vi "TEST User Events XControl.vi"() -> ()   [LabVIEW 2011]
doc: "This tests and XControl that implements the generation of User Events in an X Control that are then passed to the parent VI to be handled with dynamic registration.\n\nAAL 9/09"
uses:
  XControlUserEvents.xctl
panel:
  in  "XControlUserEvents":string(xcontrol)
  in  "stop":bool
  out "Output":string
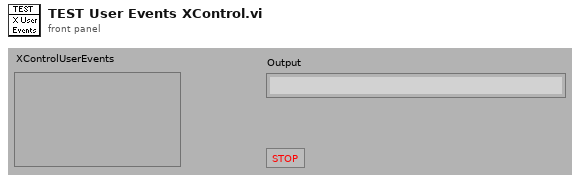
[diagram p1: front panel]
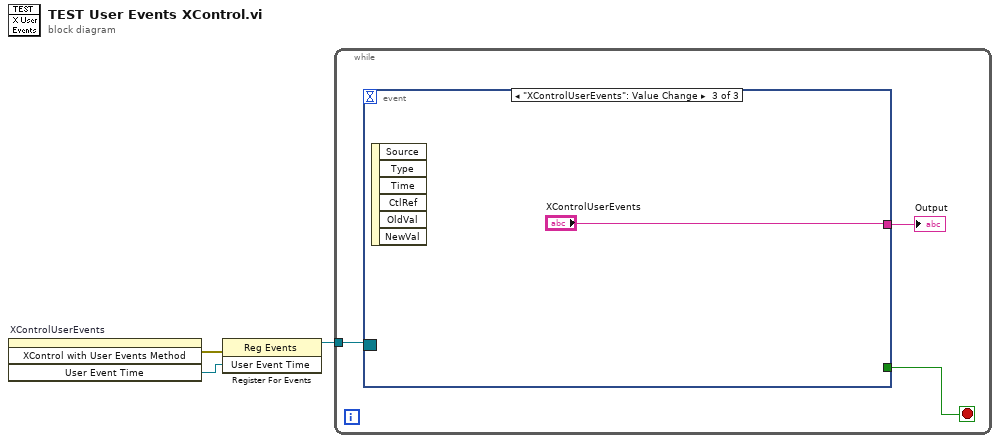
[diagram p0: block diagram]
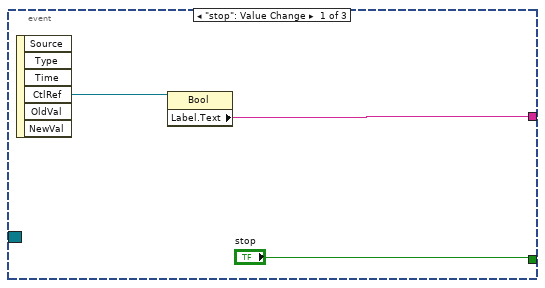
[diagram p2: hidden frame]
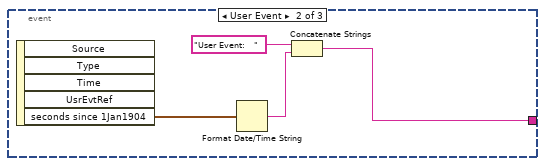
[diagram p3: hidden frame]
diagram:
  n1 = invoke on="XControlUserEvents" class="XControlUserEvents (strict)" method="XControl with User Events Method"() -> (error out=w3:errorcluster, "User Event Time"=w2:refnum<user-event>)  [unwired: 4 in, 2 out]
  n2 = register-events(error in=w3, w2) -> (reference out=w1:refnum<event-registration>)  [unwired: 1 in, 1 out]
  n3 = while {
    tunnel: w1 -> [w5]
    stop <- w6 stop-if-true
    n4 = event shown="[2] \"XControlUserEvents\": Value Change" {
      selector: w5 -> [_ _ _]
      dyn-events: _ -> [_ _ _]
      timeout: _ -> [_ _ _]
      tunnel: ["stop" _ _] -> w6
      tunnel: [w7 w10 "XControlUserEvents"] -> w4
      event "stop": Value Change {
        n5 = event-data() -> ("CtlRef"=w8:refnum<vi>)  [unwired: 1 in, 5 out]
        n6 = property class="Bool"(reference=w8) -> ("Label.Text"=w7:string)  [unwired: 1 in, 2 out]
      }
      event User Event {
        n7 = event-data() -> ("seconds since 1Jan1904"=w12:timestamp)  [unwired: 1 in, 4 out]
        n8 = Format Date/Time String(seconds (now)=w12) -> (date/time string=w11:string)  [unwired: 2 in]
        n9 = Concatenate Strings("User Event:   " ("string"), w11) -> (w10:string)
      }
      event "XControlUserEvents": Value Change {
        n10 = event-data() -> ()  [unwired: 1 in, 6 out]
      }
    }
    "Output" <- w4
  }
